vi "email_stopWorker.vi"(8 "entrée d'erreur (pas d'erreur)":errorcluster) -> (0 "sortie d'erreur":errorcluster)   [LabVIEW 2020]
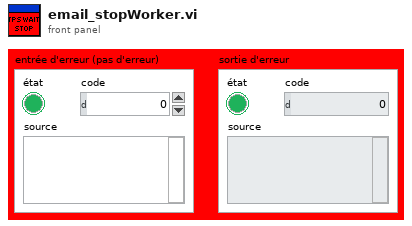
[diagram p1: front panel]
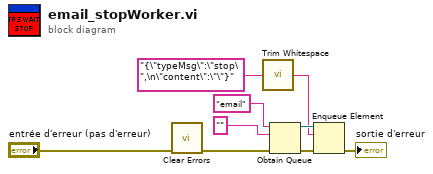
[diagram p0: block diagram]
diagram:
  n1 = call <vilib>:"Clear Errors.vi"("error in (no error)"="entrée d'erreur (pas d'erreur)") -> ("error out"=w1:errorcluster)  [unwired: 5 in, 1 out]
  n2 = call <vilib>:"Trim Whitespace.vi"("string"="{\"typeMsg\":\"stop\",\n\"content\":\"\"}" ("chaîne de format")) -> ("trimmed string"=w4:string)  [unwired: 1 in]
  n3 = Obtain Queue(name (unnamed)="email" ("nom (aucun)"), element data type="" ("nom (aucun)"), error in (no error)=w1) -> (queue out=w5:refnum<queue>, error out=w3:errorcluster)  [unwired: 2 in, 1 out]
  n4 = Enqueue Element(queue=w5, element=w4, error in (no error)=w3) -> (error out=→"sortie d'erreur":errorcluster)  [unwired: 1 in, 2 out]
